vi "BRig_RT__Case_Exp__comm_tcp__data_other.vi"(7 "input_strState":string, 8 "input_strAccum":string, 9 "input_error":errorcluster, 10 "input_hTCP":refnum<k5>, 11 "input_I_connected_TCP":bool) -> (0 "output_strAccum":string, 1 "output_error":errorcluster, 2 "output_hTCP":refnum<k5>, 3 "output_I_connect_TCP":bool)   [LabVIEW 2014]
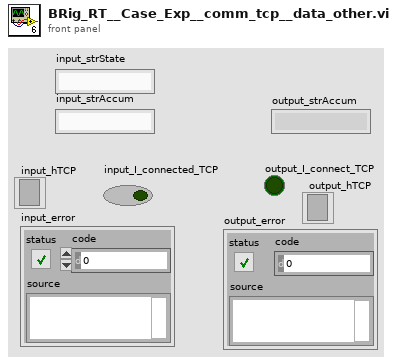
[diagram p1: front panel]
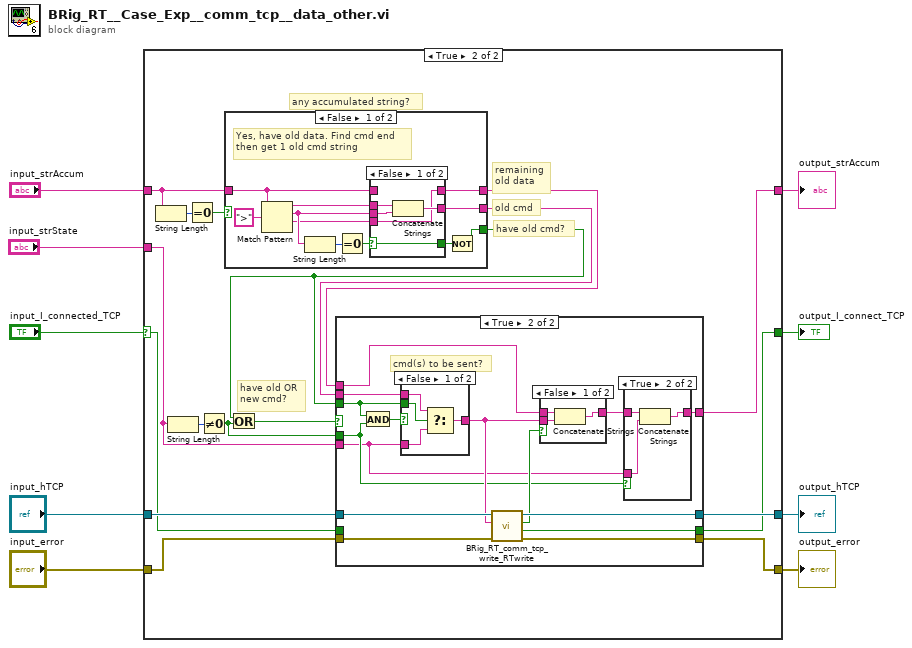
[diagram p0: block diagram]
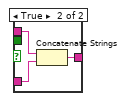
[diagram p6: hidden frame]
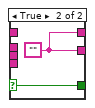
[diagram p7: hidden frame]
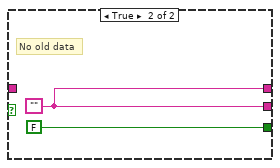
[diagram p8: hidden frame]
diagram:
  n1 = case shown="True" "input_I_connected_TCP" {
    selector: "input_I_connected_TCP" -> [w11 w14]
    tunnel: "input_hTCP" -> [w13 w30]
    tunnel: "input_error" -> [w12 w29]
    tunnel: [w13 w18] -> w3
    tunnel: [w12 w17] -> w2
    tunnel: [w11 w16] -> w4
    tunnel: "input_strAccum" -> [w10 w26]
    tunnel: [w10 w15] -> w5
    tunnel: "input_strState" -> [_ w20]
    frame False {
    }
    frame True {
      # "have old OR\nnew cmd?"
      # "remaining\nold data"
      # "old cmd"
      # "have old cmd?"
      # "any accumulated string?"
      n2 = String Length(string=w26) -> (length=w28:i32)
      n3 = String Length(string=w20) -> (length=w25:i32)
      n4 = Equal To 0?(x=w28) -> (x = 0?=w27:bool)
      n5 = Not Equal To 0?(x=w25) -> (x != 0?=w19:bool)
      n6 = case shown="False" w27 {
        tunnel: w26 -> [w72 _]
        tunnel: [w68 w84] -> w22
        tunnel: [w67 w84] -> w21
        tunnel: [w65 FALSE] -> w23
        frame False {
          # "Yes, have old data. Find cmd end\nthen get 1 old cmd string"
          n7 = Match Pattern(string=w72, regular expression=">" ("search string/char (-)")) -> (before substring=w71:string, match substring=w70:string, after substring=w69:string)  [unwired: 1 in, 1 out]
          n8 = String Length(string=w70) -> (length=w75:i32)
          n9 = Equal To 0?(x=w75) -> (x = 0?=w73:bool)
          n10 = case shown="False" w73 {
            selector: w73 -> [w76 w81]
            tunnel: w72 -> [_ _]
            tunnel: w71 -> [w80 _]
            tunnel: w70 -> [w79 _]
            tunnel: w69 -> [w77 _]
            tunnel: [w78 w82] -> w68
            tunnel: [w77 w82] -> w67
            tunnel: [w76 w81] -> w66
            frame False {
              n11 = Concatenate Strings(w80, w79) -> (w78:string)
            }
            frame True {
              w82 = ""
            }
          }
          n12 = Not(x=w66) -> (.not. x?=w65:bool)
        }
        frame True {
          w84 = ""
          # "No old data"
        }
      }
      n13 = Or(x=w23, y=w19) -> (x .or. y?=w24:bool)
      n14 = case shown="True" w24 {
        tunnel: w30 -> [w34 w46]
        tunnel: w29 -> [w33 w45]
        tunnel: w23 -> [_ w47]
        tunnel: w22 -> [_ w48]
        tunnel: w21 -> [w31 w39]
        tunnel: w20 -> [_ w37]
        tunnel: w19 -> [_ w38]
        tunnel: [w34 w44] -> w18
        tunnel: [w33 w43] -> w17
        tunnel: [w32 w42] -> w16
        tunnel: [w31 w35] -> w15
        tunnel: w14 -> [w32 _]
        frame False {
        }
        frame True {
          # "cmd(s) to be sent?"
          n15 = And(x=w47, y=w38) -> (x .and. y?=w49:bool)
          n16 = case shown="False" w49 {
            tunnel: w48 -> [w60 w64]
            tunnel: w37 -> [w59 w63]
            tunnel: w47 -> [w61 _]
            tunnel: [w58 w62] -> w40
            frame False {
              n17 = Select(t=w60, s=w61, f=w59) -> (s? t:f=w58:string)
            }
            frame True {
              n18 = Concatenate Strings(w64, w63) -> (w62:string)
            }
          }
          n19 = call "BRig_RT_comm_tcp_write_RTwrite.vi"("input_error"=w45, "input_packet"=w40, "input_hTCP"=w46) -> ("output_error"=w43:errorcluster, "output_I_NotDisconnected"=w42:bool, "output_I_write"=w41:bool, "output_hTCP"=w44:refnum<k5>)  [unwired: 5 in]
          n20 = case shown="False" w41 {
            tunnel: w40 -> [w55 _]
            tunnel: w39 -> [w56 w57]
            tunnel: [w54 w57] -> w36
            frame False {
              n21 = Concatenate Strings(w56, w55) -> (w54:string)
            }
            frame True {
            }
          }
          n22 = case shown="True" w38 {
            tunnel: w37 -> [_ w53]
            tunnel: w36 -> [w50 w52]
            tunnel: [w50 w51] -> w35
            frame False {
            }
            frame True {
              n23 = Concatenate Strings(w52, w53) -> (w51:string)
            }
          }
        }
      }
    }
  }
  "output_strAccum" <- w5
  "output_I_connect_TCP" <- w4
  "output_hTCP" <- w3
  "output_error" <- w2
